vi "LEDData.vi"() -> ()   [LabVIEW 2017]
uses:
  Implements/TypeDefs/IntakeState.ctl
  Implements/Arm/TypeDefs/ArmTargetPosition.ctl
panel:
  in  "ArmTargetPosition":T1
  in  "IntakeState":T2
  in  "ScaleArmHeight":dbl
  in  "ArmHeight":dbl
  in  "Climbing":bool
  in  "Win":bool
  in  "LED Auto Mode":T3(ring)
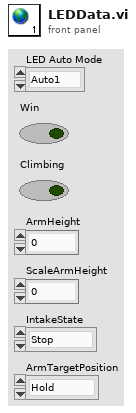
[diagram p1: front panel]
types:
  T1 = typedef "ArmTargetPosition.ctl" = enum16{"Hold", "Switch", "Scale Low", "Scale High", "Climb", "Back Place"}
  T2 = typedef "IntakeState.ctl" = enum16{"Stop", "Forward", "Reverse", "Forward Open"}
  T3 = enum16{"Auto1", "Auto2", "Auto3", "Auto4", "Auto5", "Auto6"}
diagram:
